vi "FdxCmdRxEDECreatePortCvi.vi"(8 "error in":errorcluster, 9 "EDERxDescription":T1, 10 "UdpDescription":T2 {"PortType" items=["FDX_UDP_SAMPLING", "FDX_UDP_QUEUING"]}, 11 "InstrumentHandle":u32) -> (0 "error out":errorcluster, 1 "EDEPortHandle":u32, 3 "InstrumentHandle":u32)   [LabVIEW 2020, in "AIM664LV.lvlib"]
doc: "This function is used to create and configure a new EDE enabled UDP port."
uses:
  AIM664LV.lvlib
  AFDX_LibraryAdmin/FdxGlobalDllPath.vi
panel:
  # "Inputs"
  # "Outputs"
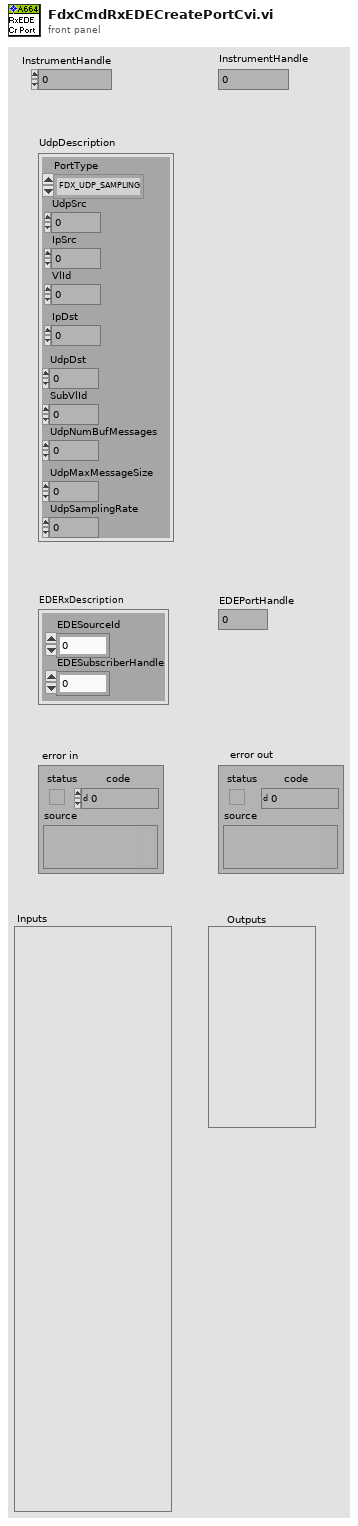
[diagram p1: front panel]
types:
  T1 = cluster{"EDESourceId":u32, "EDESubscriberHandle":u32}
  T2 = cluster{"PortType":u32, "UdpSrc":u32, "IpSrc":u32, "VlId":u32, "IpDst":u32, "UdpDst":u32, "SubVlId":u32, "UdpNumBufMessages":u32, "UdpMaxMessageSize":u32, "UdpSamplingRate":u32}
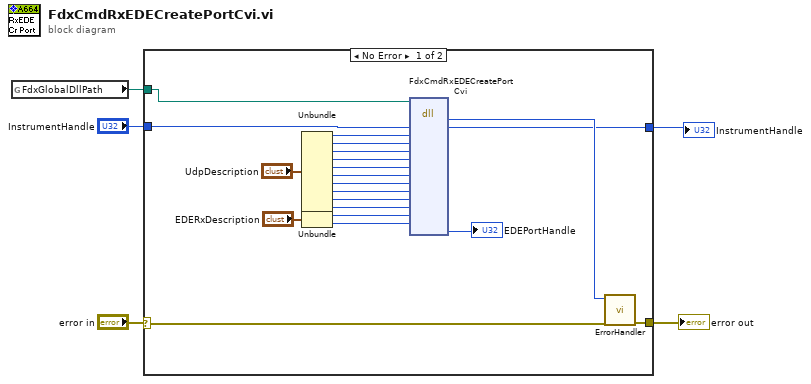
[diagram p0: block diagram]
diagram:
  n1 = global read "FdxGlobalDllPath.vi" "FdxGlobalDllPath"() -> (w3:path)
  n2 = case shown="No Error" "error in" {
    selector: "error in" -> [w25 w28]
    tunnel: [w26 w28] -> w5
    tunnel: w3 -> [w8 _]
    tunnel: "InstrumentHandle" -> [w7 w27]
    tunnel: [w6 w27] -> w1
    frame No Error {
      n3 = Unbundle("UdpDescription") -> ("PortType"=w20:u32, "UdpSrc"=w19:u32, "IpSrc"=w18:u32, "VlId"=w17:u32, "IpDst"=w16:u32, "UdpDst"=w15:u32, "SubVlId"=w14:u32, "UdpNumBufMessages"=w13:u32, "UdpMaxMessageSize"=w12:u32, "UdpSamplingRate"=w11:u32)
      n4 = Unbundle("EDERxDescription") -> ("EDESourceId"=w10:u32, "EDESubscriberHandle"=w9:u32)
      n5 = dll-call lib="aim_fdx.19.dll" fn="FdxCmdRxEDECreatePortCvi"(path in=w8, "InstrumentHandle"=w7, "PortType"=w20, "UdpSrc"=w19, "IpSrc"=w18, "VlId"=w17, "IpDst"=w16, "UdpDst"=w15, "SubVlId"=w14, "UdpNumBufMessages"=w13, "UdpMaxMessageSize"=w12, "UdpSamplingRate"=w11, "EDESourceId"=w10, "EDESubscriberHandle"=w9) -> ("status"=w24:i32, "InstrumentHandle"=w6:u32, "EDEPortHandle"=→"EDEPortHandle":u32)  [unwired: 14 in, 3 out]
      n6 = call "ErrorHandler.vi"("error in"=w25, "AIM Error"=w24) -> ("error out"=w26:errorcluster)  [unwired: 9 in]
    }
    frame Error {
    }
  }
  "error out" <- w5
  "InstrumentHandle" <- w1
